vi "sv_Check Range Parameters.vi"(8 "error in (no error)":errorcluster, 10 "fs":dbl=10.0, 11 "harmonic range":cluster{"start":dbl, "stop":dbl}={"start"=-1.0, "stop"=-1.0} {"stop" format="%.2f"; "start" format="%.2f"}) -> (0 "error out":errorcluster, 2 "fs out":dbl=10.0, 3 "harmonic range out":cluster{"start":dbl, "stop":dbl}={"start"=-1.0, "stop"=-1.0} {"stop" format="%.2f"; "start" format="%.2f"})   [LabVIEW 2017, in "SoundVib_ContSweptSine.lvlib"]
uses:
  <vilib>/addons/Sound and Vibration/svt_Continuous Swept Sine/SoundVib_ContSweptSine.lvlib
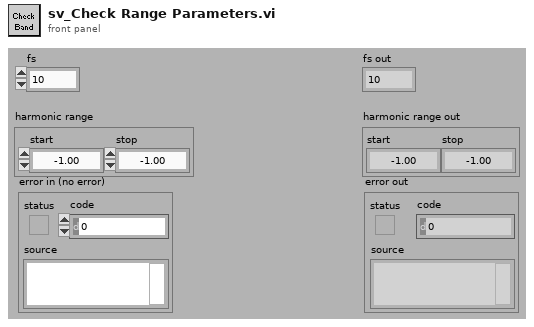
[diagram p1: front panel]
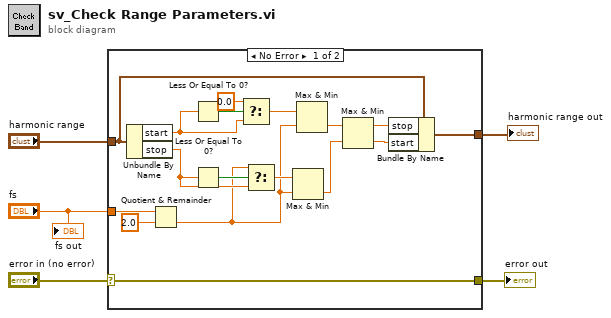
[diagram p0: block diagram]
diagram:
  n1 = case shown="No Error" "error in (no error)" {
    selector: "error in (no error)" -> [w12 w24]
    tunnel: "fs" -> [w19 _]
    tunnel: "harmonic range" -> [w15 w23]
    tunnel: [w12 w24] -> w3
    tunnel: [w11 w23] -> w1
    frame No Error {
      n2 = Unbundle By Name(w15) -> ("start"=w21:dbl, "stop"=w16:dbl)
      n3 = Quotient & Remainder(x=w19, y=2.0) -> (floor(x/y)=w7:dbl)  [unwired: 1 out]
      n4 = Less Or Equal To 0?(x=w21) -> (x <= 0?=w22:bool)
      n5 = Less Or Equal To 0?(x=w16) -> (x <= 0?=w17:bool)
      n6 = Select(t=0.0, s=w22, f=w21) -> (s? t:f=w10:dbl)
      n7 = Select(t=w7, s=w17, f=w16) -> (s? t:f=w8:dbl)
      n8 = Max & Min(x=w8, y=w7) -> (min(x,y)=w6:dbl)  [unwired: 1 out]
      n9 = Max & Min(x=w10, y=w7) -> (min(x,y)=w9:dbl)  [unwired: 1 out]
      n10 = Max & Min(x=w9, y=w6) -> (max(x,y)=w14:dbl, min(x,y)=w13:dbl)
      n11 = Bundle By Name(cluster=w15, "stop"=w14, "start"=w13) -> (w11:cluster{"start":dbl, "stop":dbl})
    }
    frame Error {
    }
  }
  "error out" <- w3
  "harmonic range out" <- w1
  "fs out" <- "fs"
